vi "SVL Get dB Reference (N Ch).vi"(8 "error in (no error)":errorcluster, 11 "scaled signals [EU]":waveform(dbl)[](array[waveform])=[{"t0"=timestamp(0 s since 1904-01-01), "dt"=0.0, "Y"=[]}]) -> (0 "error out":errorcluster, 2 "dB references [EU]":dbl[](array[numeric]) format="%^.1e", 3 "scaled signals [EU]":waveform(dbl)[](array[waveform]))   [LabVIEW 2017]
doc: "Returns the dB reference stored in the waveform attributes of the scaled signal input. The dB reference is set by the DAQ Assistant for Sound Pressure and Acceleration tasks, the SVL Scale Voltage to EU VI, and the SVL Set dB Reference VI. The dB reference is used for all downstream conversions to dB. Wire data to the <B>scaled signal [EU]</B> input to determine the polymorphic instance to use or manually select the instance."
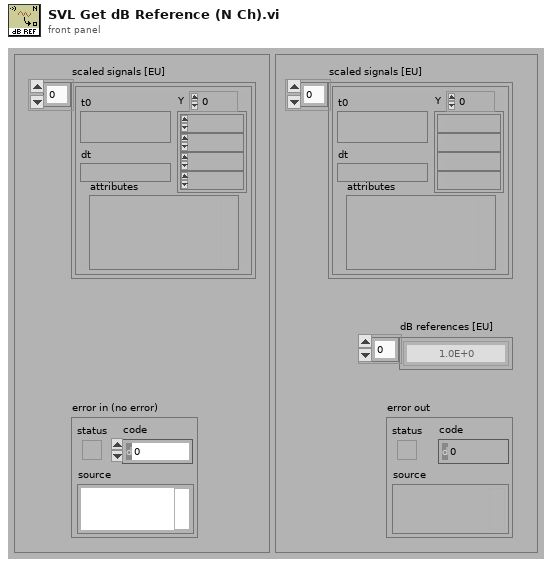
[diagram p1: front panel]
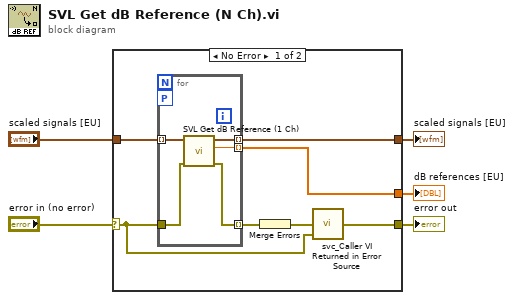
[diagram p0: block diagram]
diagram:
  n1 = case shown="No Error" "error in (no error)" {
    selector: "error in (no error)" -> [w9 w19]
    tunnel: "scaled signals [EU]" -> [w8 w18]
    tunnel: [w12 w19] -> w4
    tunnel: [w11 w18] -> w3
    tunnel: [w7 _] -> w1
    frame No Error {
      n2 = for {
        tunnel: w8 -> [w17] mode=indexing
        tunnel: [w16] -> w11 mode=indexing
        tunnel: [w13] -> w7 mode=indexing
        tunnel: w9 -> [w14]
        tunnel: [w15] -> w10 mode=indexing
        workers-P: _ -> [_]
        n3 = call <vilib>:"SVL Get dB Reference (1 Ch).vi"("error in (no error)"=w14, "scaled signal [EU]"=w17) -> ("error out"=w15:errorcluster, "dB reference [EU]"=w13:dbl, "scaled signal [EU]"=w16:waveform(dbl))  [unwired: 7 in]
      }
      n4 = Merge Errors(w10) -> (w6:errorcluster)
      n5 = call <vilib>:"svc_Caller VI Returned in Error Source.vi"("warning input to caller"=w9, "error in (no error)"=w6) -> ("error out"=w12:errorcluster)  [unwired: 3 in]
    }
    frame Error {
    }
  }
  "scaled signals [EU]" <- w3
  "error out" <- w4
  "dB references [EU]" <- w1
